vi "Get Default Encoding Name.vi"(8 "错误输入（无错误）":errorcluster) -> (0 "错误输出":errorcluster, 3 "EncodingName":string)   [LabVIEW 2012, in "Encoding.lvlib"]
uses:
  Encoding.lvlib
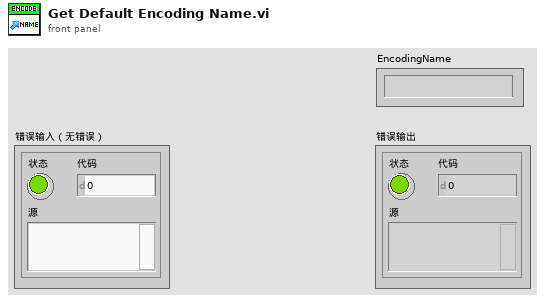
[diagram p1: front panel]
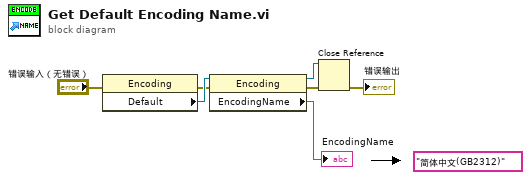
[diagram p0: block diagram]
diagram:
  (unwired) "简体中文(GB2312)" ("EncodingName")
  n1 = property class="Encoding"(error in="错误输入（无错误）") -> (error out=w5:errorcluster, "Default"=w6:refnum<k24>)  [unwired: 1 in, 1 out]
  n2 = property class="Encoding"(reference=w6, error in=w5) -> (reference out=w2:refnum<k24>, error out=w3:errorcluster, "EncodingName"=→"EncodingName":string)
  n3 = Close Reference(reference=w2, error in (no error)=w3) -> (error out=→"错误输出":errorcluster)
